vi "Page_Source_Get_Inclusion_Types.vi"() -> (3 "supportedFunctions":T1)   [LabVIEW 2020, in "AB_EXE.lvlib"]
uses:
  <vilib>/AppBuilder/AB_Classes/EXE/common/AB_EXE.lvlib
  <vilib>/AppBuilder/AB_Source_Inclusion.ctl
  <resource>/Framework/Providers/Builds/AppBuilder/AB_UI_Page_Source_Files_supportedFunctions.ctl
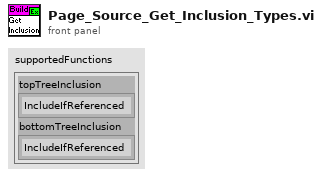
[diagram p1: front panel]
types:
  T1 = typedef "AB_UI_Page_Source_Files_supportedFunctions.ctl" = cluster{"topTreeInclusion":T2, "bottomTreeInclusion":T2}
  T2 = typedef "AB_Source_Inclusion.ctl" = enum16{"IncludeIfReferenced", "Include", "Exclude", "TopLevel"}
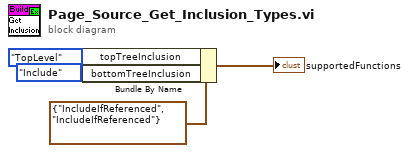
[diagram p0: block diagram]
diagram:
  n1 = Bundle By Name(cluster=T1 {"topTreeInclusion"=enum."IncludeIfReferenced", "bottomTreeInclusion"=enum."IncludeIfReferenced"} ("supportedFunctions"), "topTreeInclusion"=AB_Source_Inclusion."TopLevel", "bottomTreeInclusion"=AB_Source_Inclusion."Include") -> (→"supportedFunctions":T1)
